vi "Run Runnable.vi"(8 "error in (no error)":errorcluster, 10 "Runnable":refnum<class "Runnable.lvclass">, 11 "Test Runner":refnum<class "Single Thread Test Runner.lvclass">) -> (0 "error out":errorcluster)   [LabVIEW 2020, in "Single Thread Test Runner.lvclass"]
uses:
  Single Thread Test Runner.lvclass
  Run/Runnable.lvclass
  Execute.vi
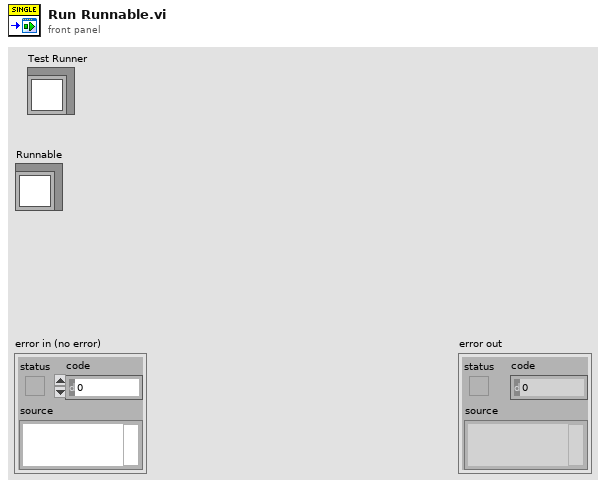
[diagram p1: front panel]
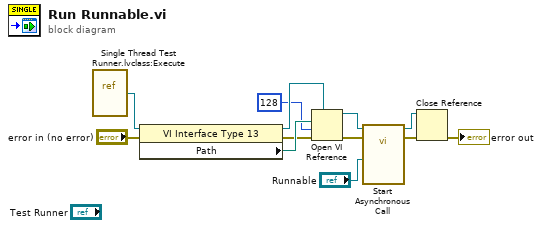
[diagram p0: block diagram]
diagram:
  n1 = vi-ref "Single Thread Test Runner.lvclass:Execute.vi"() -> (w12:refnum<vi>)
  n2 = property class="VI Interface Type 13"(reference=w12, error in="error in (no error)") -> (reference out=w10:refnum<vi>, error out=w9:errorcluster, "Path"=w11:path)
  n3 = Open VI Reference(type specifier VI Refnum (for type only)=w10, vi path=w11, options=128, error in (no error)=w9) -> (vi reference=w7:refnum<vi>, error out=w6:errorcluster)  [unwired: 2 in]
  n4 = call-by-ref "Start Asynchronous Call"(reference=w7, error in=w6, "Test Runner V2 in"="Runnable") -> (reference out=w5:refnum<vi>, error out=w4:errorcluster)  [unwired: 11 in]
  n5 = Close Reference(reference=w5, error in (no error)=w4) -> (error out=→"error out":errorcluster)
